vi "Protocol.Address Lookup Table Action.vi"(7 "Action":T2, 8 "error in (no error)":errorcluster, 9 "Address":u8, 10 "Data":T1 {"Name" format="%.0x"}, 11 "ref in":T3) -> (0 "error out":errorcluster {"code" min=0 max=0}, 1 "Found?":bool, 2 "Data":T1 {"Name" format="%.0x"}, 4 "All Data":T1[](array[typedef]) {"Name" format="%.0x"})   [LabVIEW 2015, in "J1939 Addon Engine.lvlib"]
uses:
  J1939 Addon Engine.lvlib
  Types/Protocol.Address Table Reference.ctl
  Shared/Types/Address Lookup Table Data.ctl
  Types/Protocol.Address Lookup Table Action.ctl
  Shared/J1939 Addon Shared.lvlib
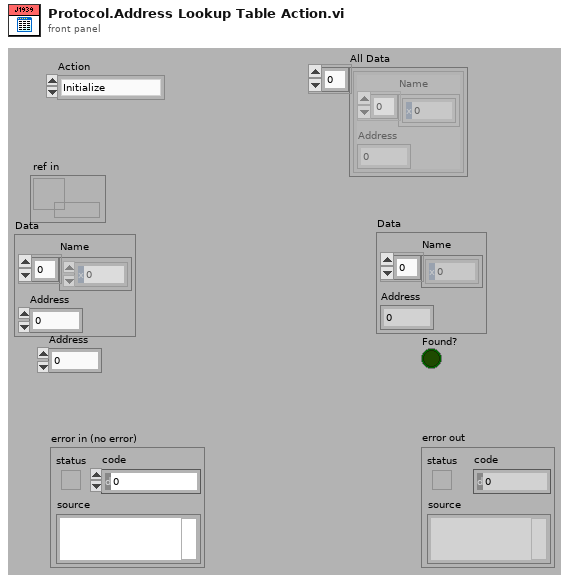
[diagram p1: front panel]
types:
  T1 = typedef "J1939 Addon Shared.lvlib/Address Lookup Table Data.ctl" = cluster{"Name":u8[], "Address":u8}
  T2 = typedef "J1939 Addon Engine.lvlib/Protocol.Address Lookup Table Action.ctl" = enum16{"Initialize", "Add", "Get", "Remove", "Get All"}
  T3 = typedef "J1939 Addon Engine.lvlib/Protocol.Address Table Reference.ctl" = refnum<data-value>
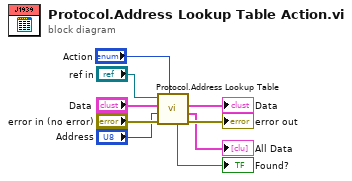
[diagram p0: block diagram]
diagram:
  n1 = call "Protocol.Address Lookup Table.vi"("Action"="Action", "error in (no error)"="error in (no error)", "Address"="Address", "Data"="Data", "Address LUT"="ref in") -> ("error out"=→"error out":errorcluster, "All Data"=→"All Data":T1[], "Data"=→"Data":T1, "Found?"=→"Found?":bool)  [unwired: 2 in, 1 out]
